vi "Configurar.vi"(8 "error in (no error)":errorcluster, 11 "Camara in":refnum<class "Camara.lvclass">) -> (0 "error out":errorcluster, 3 "Camara out":refnum<class "Camara.lvclass">)   [LabVIEW 2020, in "Camara.lvclass"]
uses:
  Camara.lvclass
  Camara.lvclass/Camara.ctl
  Write New Image.vi
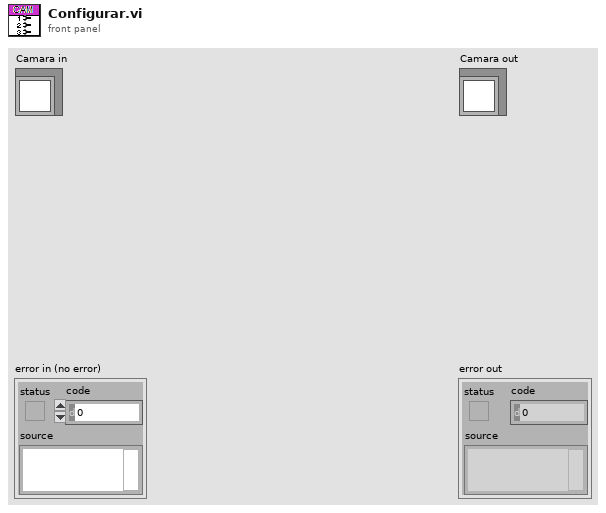
[diagram p1: front panel]
types:
  T1 = typedef "IMAQ Image.ctl" = refnum<image>
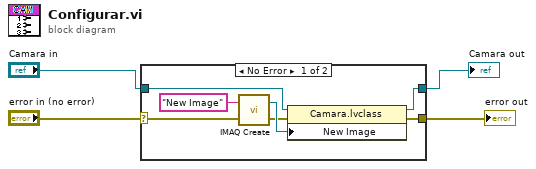
[diagram p0: block diagram]
diagram:
  n1 = case shown="No Error" "error in (no error)" {
    selector: "error in (no error)" -> [w6 w13]
    tunnel: [w11 w13] -> w3
    tunnel: [w9 w12] -> w1
    tunnel: "Camara in" -> [w10 w12]
    frame No Error {
      n2 = call "IMAQ Create"("Image Name"="New Image", "error in (no error)"=w6) -> ("New Image"=w7:T1, "error out"=w5:errorcluster)  [unwired: 3 in]
      n3 = property class="Camara.lvclass"(reference=w10, error in=w5, "New Image"=w7) -> (reference out=w9:refnum<class "Camara.lvclass">, error out=w11:errorcluster)
    }
    frame Error {
    }
  }
  "error out" <- w3
  "Camara out" <- w1
